vi "Open 44_1.vi"(7 "init":bool, 8 "error in (no error)":errorcluster, 11 "Stand in":refnum<class "Stand.lvclass">) -> (0 "error out":errorcluster, 3 "Stand out":refnum<class "Stand.lvclass">)   [LabVIEW 2019, in "Stand.lvclass"]
uses:
  Stand.lvclass
  Stand.lvclass/Stand.ctl
  Valve_2DO_2DI_class/Valve_2DO_2DI.lvclass/Valve_2DO_2DI.ctl
  Device_class/Device.lvclass/Device.ctl
  73fa1956-3950-4b5c-ac69-61251d44dc94.vi
  Device_class/GetFPGA.vi
  Valve_2DO_2DI_class/Valve_2DO_2DI.lvclass
  C:/Users/ANENKOV_V1/Desktop/src/Device_class/Device.lvclass
  FPGA_API_class/FPGA API.lvclass
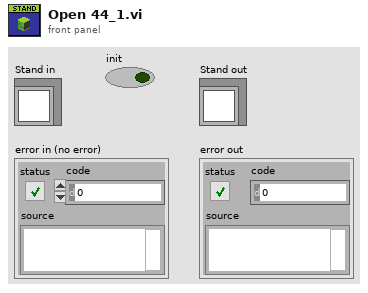
[diagram p1: front panel]
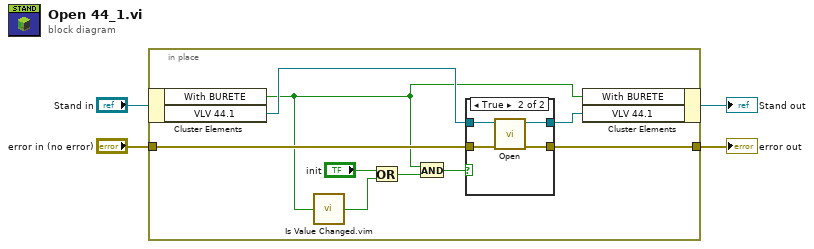
[diagram p0: block diagram]
diagram:
  n1 = in-place {
    in-place-border: "error in (no error)" -> [w12]
    in-place-border: [w10] -> w1
    n2 = in-place-cluster #1("Stand in") -> ("With BURETE"=w5:bool, "VLV 44.1"=w13:refnum<class "Valve_2DO_2DI.lvclass">)
    n3 = call "Is Value Changed.vim"("value"=w5) -> ("changed or first call?"=w9:bool)
    n4 = Or(x="init", y=w9) -> (x .or. y?=w7:bool)
    n5 = And(x=w5, y=w7) -> (x .and. y?=w6:bool)
    n6 = case shown="True" w6 {
      tunnel: w13 -> [w15 w19]
      tunnel: w12 -> [w14 w18]
      tunnel: [w15 w17] -> w11
      tunnel: [w14 w16] -> w10
      frame False {
      }
      frame True {
        n7 = call "Open.vi"("error in (no error)"=w18, "Pump_1AI_1DO_2DI in"=w19) -> ("error out"=w16:errorcluster, "Pump_1AI_1DO_2DI out"=w17:refnum<class "Valve_2DO_2DI.lvclass">)  [unwired: 8 in]
      }
    }
    n8 = in-place-cluster #1("With BURETE"=w5, "VLV 44.1"=w11) -> (→"Stand out":refnum<class "Stand.lvclass">)
  }
  "error out" <- w1
